vi "Get Visible (Label).vi"(8 "error in (no error)":errorcluster, 10 "Label":string, 11 "IContainer in":refnum<class "IContainer.lvclass">) -> (0 "error out":errorcluster, 1 "Match?":bool, 2 "Visible?":bool, 3 "IContainer out":refnum<class "IContainer.lvclass">, 4 "Item visible?":bool)   [LabVIEW 2021, in "IContainer.lvclass"]
doc: "Copyright 2018, Wiebe Walstra, wiebe@carya.nl."
uses:
  IContainer.lvclass
  IContainer.lvclass/IContainer.ctl
  IObject.lvclass
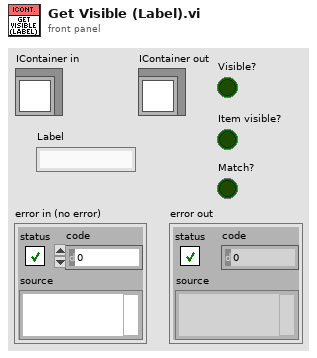
[diagram p1: front panel]
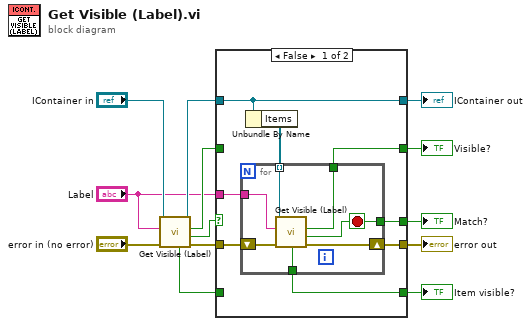
[diagram p0: block diagram]
diagram:
  n1 = call-parent "Get Visible (Label).vi"("error in (no error)"="error in (no error)", "Label"="Label", "IObject in"="IContainer in") -> ("error out"=w10:errorcluster, "Match?"=w9:bool, "Visible?"=w6:bool, "IObject out"=w3:refnum<class "IContainer.lvclass">, "Item visible?"=w4:bool)  [unwired: 4 in]
  n2 = case shown="False" w9 {
    selector: w9 -> [_ w31]
    tunnel: [w20 w30] -> w11
    tunnel: w10 -> [w21 w30]
    tunnel: [w15 w31] -> w8
    tunnel: [w14 w32] -> w7
    tunnel: w6 -> [_ w32]
    tunnel: [w16 w29] -> w5
    tunnel: w4 -> [_ w29]
    tunnel: w3 -> [w18 w33]
    tunnel: [w18 w33] -> w2
    tunnel: "Label" -> [w17 _]
    frame False {
      n3 = Unbundle By Name(w18) -> ("Items"=w19:refnum<class "IObject.lvclass">[])
      n4 = for {
        tunnel: w19 -> [w26] mode=indexing
        shift-right: [w28] -> w20
        shift-left: w21 -> [w27]
        tunnel: w17 -> [w25]
        tunnel: [w24] -> w16
        tunnel: [w22] -> w15
        tunnel: [w23] -> w14
        stop <- w22 stop-if-true
        n5 = call-dynamic "Get Visible (Label).vi"("error in (no error)"=w27, "Label"=w25, "IObject in"=w26) -> ("error out"=w28:errorcluster, "Match?"=w22:bool, "Visible?"=w23:bool, "Item visible?"=w24:bool)  [unwired: 4 in, 1 out]
      }
    }
    frame True {
    }
  }
  "error out" <- w11
  "IContainer out" <- w2
  "Visible?" <- w7
  "Item visible?" <- w5
  "Match?" <- w8
